vi "_test_RecombinatorGAOperator(binary).vi"() -> ()   [LabVIEW 2016]
uses:
  IGene/Children/Binary/_typedefs/BinaryGene_Allele.ctl
  GA Core/Genetic Operators/Recombinator/Children/N-Point Crossover.lvclass
  C:/Users/J51654/My Projects/Evolutionary Programming/GA Framework/GA Core/GA Core.lvclass
  IGene/Children/Binary/Binary Gene.lvclass
  C:/Users/J51654/My Projects/Evolutionary Programming/GA Framework/IGene/IGene.lvclass
  IGene/Children/RealVal/Real Gene.lvclass
  GA Core/Genetic Operators/Recombinator/Children/N-Point Crossover/_Typedefs/X-Point Crossover.ctl
  GA Core/Genetic Operators/Recombinator/Children/N-Point Crossover.lvclass/N-Point Crossover.ctl
  GA Core/GA Core.lvclass/GA Core.ctl
  IChromosome/IChromosome.lvclass/IChromosome.ctl
  IGene/Children/Binary/Binary Gene.lvclass/Binary Gene.ctl
  GA Core/Genetic Operators/Recombinator/Children/N-Point Crossover/Accessors/Write Number of Crossover Points.vi
  IGene/IGene.lvclass
  GA Core/GA Core.lvclass
  IChromosome/IChromosome.lvclass
panel:
  out "Parent 1 (R)":dbl[](array[numeric])
  out "Parent 2(R)":dbl[](array[numeric])
  out "Parent 1":T1[](array[typedef])
  out "Parent 2":T1[](array[typedef])
  out "Child 1 (R)":dbl[](array[numeric])
  out "Child 2 (R)":dbl[](array[numeric])
  out "Child 1":T1[](array[typedef])
  out "Child 2":T1[](array[typedef])
  in  "Recombination Rate":dbl
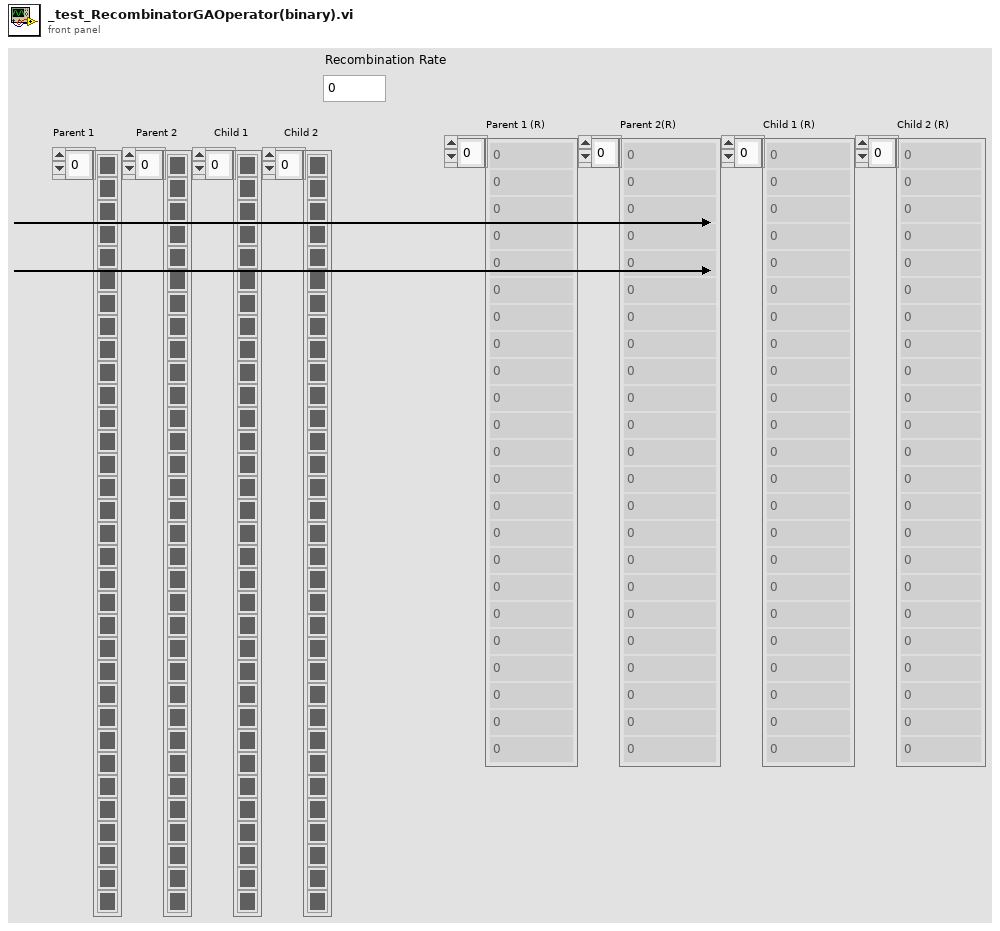
[diagram p1: front panel]
types:
  T1 = typedef "Binary Gene.lvclass/BinaryGene_Allele.ctl" = bool
  T2 = typedef "N-Point Crossover.lvclass/X-Point Crossover.ctl" = enum16{"Single-point Crossover", "Dual-point Crossover"}
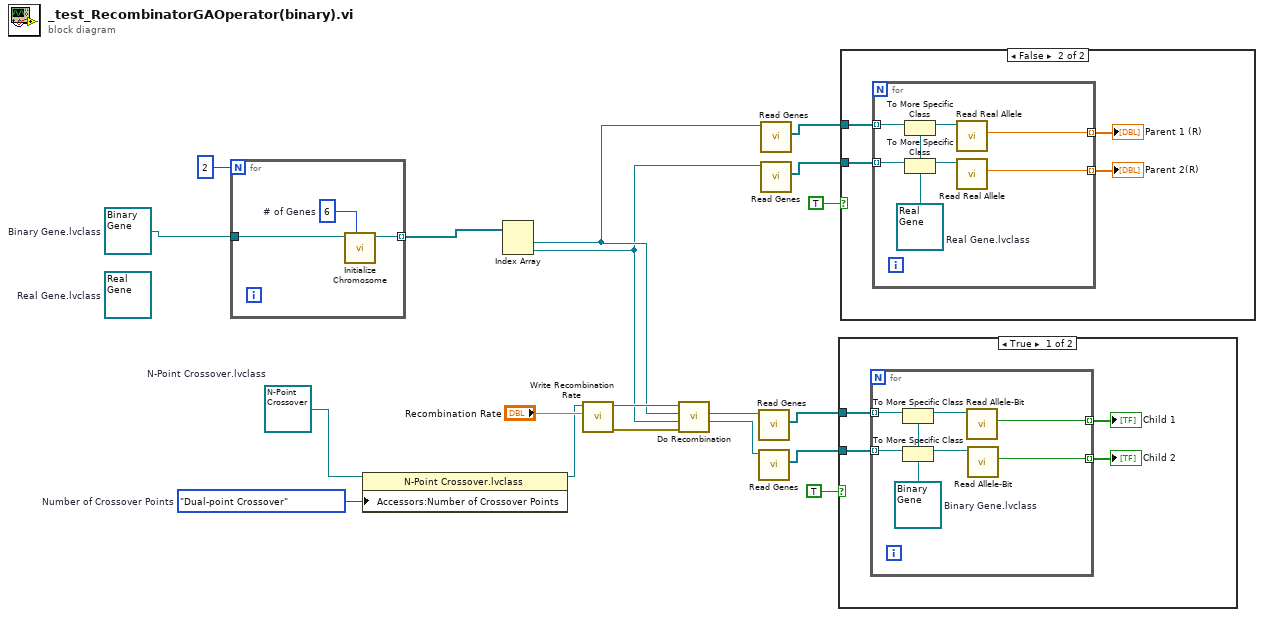
[diagram p0: block diagram]
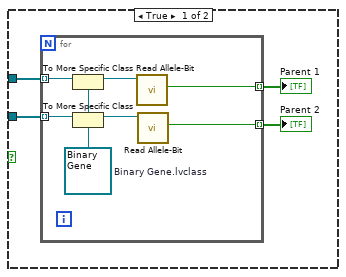
[diagram p2: hidden frame]
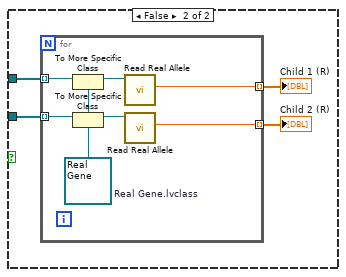
[diagram p3: hidden frame]
diagram:
  w2 = X-Point_Crossover."Dual-point Crossover"  # Number of Crossover Points
  (unwired) refnum<class "Real Gene.lvclass"> refnum  # Real Gene.lvclass
  w1 = refnum<class "Binary Gene.lvclass"> refnum  # Binary Gene.lvclass
  w4 = refnum<class "N-Point Crossover.lvclass"> refnum  # N-Point Crossover.lvclass
  n1 = for {
    N: 2 -> [_]
    tunnel: w1 -> [w21]
    tunnel: [w20] -> w16 mode=indexing
    w22 = u32 6  # # of Genes
    n2 = call "Initialize Chromosome.vi"("# of Genes"=w22, "Gene Type In"=w21) -> ("Chromosome out"=w20:refnum<class "IChromosome.lvclass">)  [unwired: 8 in, 1 out]
  }
  n3 = property class="N-Point Crossover.lvclass"(reference=w4, "Accessors:Number of Crossover Points"=w2) -> (reference out=w3:refnum<class "N-Point Crossover.lvclass">)  [unwired: 1 in, 1 out]
  n4 = Index Array(array=w16) -> (element #1=w6:refnum<class "IChromosome.lvclass">, element #2=w5:refnum<class "IChromosome.lvclass">)  [unwired: 2 in]
  n5 = call "Write Recombination Rate.vi"("Recombination Rate"="Recombination Rate", "GA Core in"=w3) -> ("error out"=w15:errorcluster, "GA Core out"=w19:refnum<class "N-Point Crossover.lvclass">)  [unwired: 8 in]
  n6 = call-dynamic "Do Recombination.vi"("error in"=w15, "IChromosome Parent B in"=w5, "IChromosome Parent A in"=w6, "N-Point Crossover in"=w19) -> ("IChromosome Child B out"=w13:refnum<class "IChromosome.lvclass">, "IChromosome Child A out"=w14:refnum<class "IChromosome.lvclass">)  [unwired: 4 in, 2 out]
  n7 = call "Read Genes.vi"("IChromosome in"=w14) -> ("Genes"=w12:refnum<class "IGene.lvclass">[])  [unwired: 8 in, 2 out]
  n8 = call "Read Genes.vi"("IChromosome in"=w13) -> ("Genes"=w11:refnum<class "IGene.lvclass">[])  [unwired: 8 in, 2 out]
  n9 = call "Read Genes.vi"("IChromosome in"=w6) -> ("Genes"=w9:refnum<class "IGene.lvclass">[])  [unwired: 8 in, 2 out]
  n10 = call "Read Genes.vi"("IChromosome in"=w5) -> ("Genes"=w8:refnum<class "IGene.lvclass">[])  [unwired: 8 in, 2 out]
  n11 = case shown="True" TRUE {
    tunnel: w12 -> [w26 w37]
    tunnel: w11 -> [w25 w36]
    frame True {
      n12 = for {
        tunnel: w26 -> [w33] mode=indexing
        tunnel: w25 -> [w30] mode=indexing
        tunnel: [w28] -> w24 mode=indexing
        tunnel: [w27] -> w23 mode=indexing
        w31 = refnum<class "Binary Gene.lvclass"> refnum  # Binary Gene.lvclass
        n13 = To More Specific Class(target class=w31, reference=w33) -> (specific class reference=w32:refnum<class "Binary Gene.lvclass">)  [unwired: 1 in, 1 out]
        n14 = To More Specific Class(target class=w31, reference=w30) -> (specific class reference=w29:refnum<class "Binary Gene.lvclass">)  [unwired: 1 in, 1 out]
        n15 = call "Read Allele-Bit.vi"("Binary Gene in"=w32) -> ("Allele-Bit"=w28:T1)  [unwired: 8 in, 2 out]
        n16 = call "Read Allele-Bit.vi"("Binary Gene in"=w29) -> ("Allele-Bit"=w27:T1)  [unwired: 8 in, 2 out]
      }
      "Child 1" <- w24
      "Child 2" <- w23
    }
    frame False {
      n17 = for {
        tunnel: w37 -> [w44] mode=indexing
        tunnel: w36 -> [w43] mode=indexing
        tunnel: [w39] -> w35 mode=indexing
        tunnel: [w38] -> w34 mode=indexing
        w42 = refnum<class "Real Gene.lvclass"> refnum  # Real Gene.lvclass
        n18 = To More Specific Class(target class=w42, reference=w44) -> (specific class reference=w41:refnum<class "Real Gene.lvclass">)  [unwired: 1 in, 1 out]
        n19 = To More Specific Class(target class=w42, reference=w43) -> (specific class reference=w40:refnum<class "Real Gene.lvclass">)  [unwired: 1 in, 1 out]
        n20 = call "Read Real Allele.vi"("Real Gene in"=w41) -> ("Real Allele"=w39:dbl)  [unwired: 8 in, 2 out]
        n21 = call "Read Real Allele.vi"("Real Gene in"=w40) -> ("Real Allele"=w38:dbl)  [unwired: 8 in, 2 out]
      }
      "Child 1 (R)" <- w35
      "Child 2 (R)" <- w34
    }
  }
  n22 = case shown="False" TRUE {
    tunnel: w9 -> [w48 w59]
    tunnel: w8 -> [w47 w58]
    frame True {
      n23 = for {
        tunnel: w48 -> [w55] mode=indexing
        tunnel: w47 -> [w52] mode=indexing
        tunnel: [w50] -> w46 mode=indexing
        tunnel: [w49] -> w45 mode=indexing
        w53 = refnum<class "Binary Gene.lvclass"> refnum  # Binary Gene.lvclass
        n24 = To More Specific Class(target class=w53, reference=w55) -> (specific class reference=w54:refnum<class "Binary Gene.lvclass">)  [unwired: 1 in, 1 out]
        n25 = To More Specific Class(target class=w53, reference=w52) -> (specific class reference=w51:refnum<class "Binary Gene.lvclass">)  [unwired: 1 in, 1 out]
        n26 = call "Read Allele-Bit.vi"("Binary Gene in"=w54) -> ("Allele-Bit"=w50:T1)  [unwired: 8 in, 2 out]
        n27 = call "Read Allele-Bit.vi"("Binary Gene in"=w51) -> ("Allele-Bit"=w49:T1)  [unwired: 8 in, 2 out]
      }
      "Parent 1" <- w46
      "Parent 2" <- w45
    }
    frame False {
      n28 = for {
        tunnel: w59 -> [w66] mode=indexing
        tunnel: w58 -> [w65] mode=indexing
        tunnel: [w61] -> w57 mode=indexing
        tunnel: [w60] -> w56 mode=indexing
        w64 = refnum<class "Real Gene.lvclass"> refnum  # Real Gene.lvclass
        n29 = To More Specific Class(target class=w64, reference=w66) -> (specific class reference=w63:refnum<class "Real Gene.lvclass">)  [unwired: 1 in, 1 out]
        n30 = To More Specific Class(target class=w64, reference=w65) -> (specific class reference=w62:refnum<class "Real Gene.lvclass">)  [unwired: 1 in, 1 out]
        n31 = call "Read Real Allele.vi"("Real Gene in"=w63) -> ("Real Allele"=w61:dbl)  [unwired: 8 in, 2 out]
        n32 = call "Read Real Allele.vi"("Real Gene in"=w62) -> ("Real Allele"=w60:dbl)  [unwired: 8 in, 2 out]
      }
      "Parent 1 (R)" <- w57
      "Parent 2(R)" <- w56
    }
  }
